vi "Cross Spectrum (Real-Im).vi"(0 "time signal X":waveform(dbl), 1 "restart averaging (F)":bool, 2 "window parameter":dbl=nan, 5 "time signal Y":waveform(dbl), 7 "window":T2=1 items=["Rectangle"=0, "Hanning"=1, "Hamming"=2, "Blackman-Harris"=3, "Exact Blackman"=4, "Blackman"=5, "Flat Top"=6, "4 Term B-Harris "=7, "7 Term B-Harris"=8, "Low Sidelobe"=9, "Blackman Nuttall"=11, "Triangle"=30, "Bartlett-Hanning"=31, "Bohman"=32, "Parzen"=33, "Welch"=34, "Kaiser"=60, "Dolph-Chebyshev"=61, "Gaussian"=62], 11 "error in (no error)":errorcluster, 12 "averaging parameters":T3={"averaging mode"=enum."No averaging", "weighting mode"=enum."Exponential", "number of averages"=10} {"number of averages" min=1}) -> (3 "averaging done":bool, 4 "real part":cluster{"f0":dbl, "df":dbl, "real part":dbl[]} {"real part" format="%.2p"; "f0" format="%0.2p"; "df" format="%0.2p"}, 6 "imaginary part":T1 {"imaginary part" format="%.2p"; "f0" format="%0.2p"; "df" format="%0.2p"}, 10 "averages completed":dbl, 15 "error out":errorcluster)   [LabVIEW 2020, in "NI_MAPro.lvlib"]
doc: "Computes the averaged cross power spectrum of the input signals. Results are returned as real and imaginary parts."
uses:
  NI_MAPro.lvlib
  windowTd.ctl
  NI_AALPro.lvlib
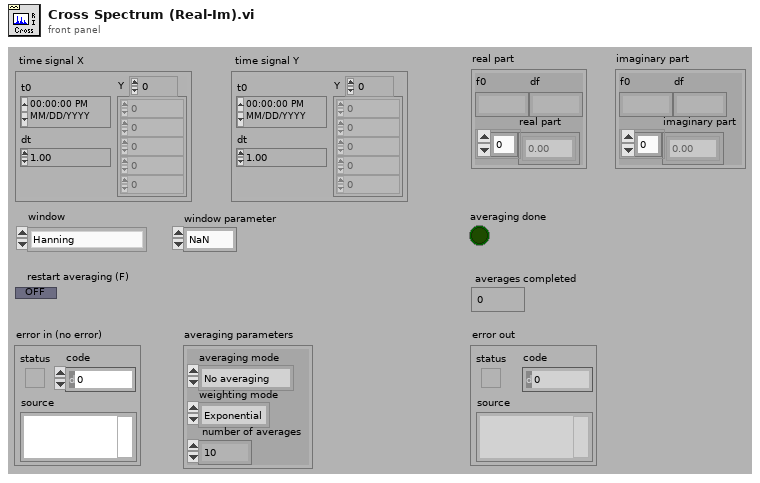
[diagram p1: front panel]
types:
  T1 = cluster{"f0":dbl, "df":dbl, "imaginary part":dbl[]}
  T2 = typedef "NI_AALPro.lvlib/windowTd.ctl" = u32
  T3 = cluster{"averaging mode":enum16{"No averaging", "Vector averaging", "RMS averaging", "Peak hold"}, "weighting mode":enum16{"Linear", "Exponential"}, "number of averages":u32}
  T4 = enum16{"No averaging", "Vector averaging", "RMS averaging", "Peak hold"}
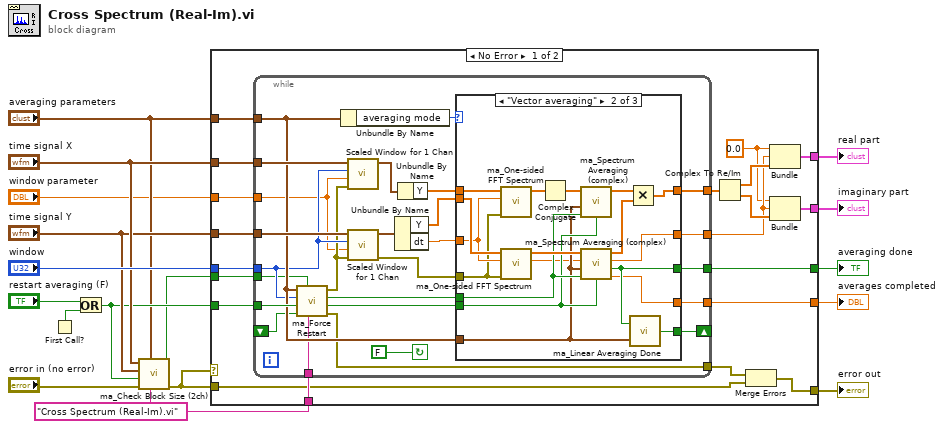
[diagram p0: block diagram]
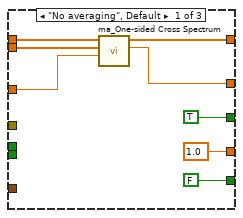
[diagram p2: hidden frame]
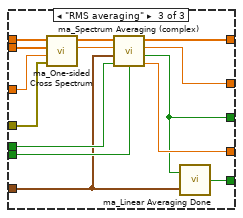
[diagram p3: hidden frame]
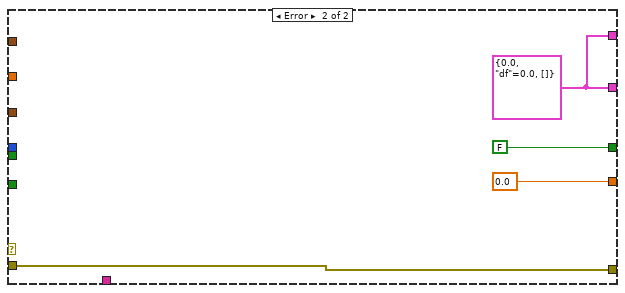
[diagram p4: hidden frame]
diagram:
  w3 = "Cross Spectrum (Real-Im).vi" ("caller VI name")
  n1 = First Call?() -> (First Call?: T/F=w7:bool)
  n2 = Or(x="restart averaging (F)", y=w7) -> (x .or. y?=w8:bool)
  n3 = call "ma_Check Block Size (2ch).vi"("caller VI name"=w3, "averaging parameters"="averaging parameters", "error in"="error in (no error)", "restart averaging (F)"=w8, "time signal Y"="time signal Y", "time signal X"="time signal X") -> ("error out"=w9:errorcluster, "force restart averaging"=w2:bool)  [unwired: 4 out]
  n4 = case shown="No Error" w9 {
    tunnel: "averaging parameters" -> [w37 _]
    tunnel: [w35 0.0 ("averages completed")] -> w17
    tunnel: "time signal X" -> [w34 _]
    tunnel: "time signal Y" -> [w33 _]
    tunnel: "window" -> [w32 _]
    tunnel: [w31 FALSE ("averaging done")] -> w15
    tunnel: w8 -> [w30 _]
    tunnel: [w23 w107] -> w14
    tunnel: w9 -> [w20 w107]
    tunnel: [w25 w104] -> w5
    tunnel: [w24 w104] -> w4
    tunnel: w3 -> [w21 _]
    tunnel: w2 -> [w19 _]
    tunnel: "window parameter" -> [w18 _]
    frame No Error {
      w26 = 0.0
      n5 = while {
        tunnel: w21 -> [w40]
        tunnel: [w41] -> w22
        tunnel: w30 -> [w55]
        shift-left: _ -> [w53]
        shift-right: [w57] -> _
        tunnel: [w58] -> w31
        tunnel: w32 -> [w45]
        tunnel: w33 -> [w59]
        tunnel: w34 -> [w60]
        tunnel: [w51] -> w27
        tunnel: [w61] -> w35
        tunnel: [w62] -> w36
        tunnel: w37 -> [w54]
        tunnel: w19 -> [w39]
        tunnel: w18 -> [w38]
        stop <- FALSE continue-if-true
        n6 = call "ma_Force Restart.vi"("caller VI name"=w40, "force restart averaging in"=w39, "linear averaging done"=w53, "restart averaging (F)"=w55, "window"=w45, "averaging parameters"=w54) -> ("error out"=w41:errorcluster, "retrieve last spectrum"=w42:bool, "force restart averaging"=w43:bool, "skip processing"=w44:errorcluster)  [unwired: 2 out]
        n7 = Unbundle By Name(w54) -> ("averaging mode"=w63:T4)
        n8 = call "Scaled Window for 1 Chan.vi"("error in (no error)"=w44, "window parameter"=w38, "window"=w45, "signal in"=w60) -> ("signal out"=w50:waveform(dbl))  [unwired: 5 in, 2 out]
        n9 = call "Scaled Window for 1 Chan.vi"("error in (no error)"=w44, "window parameter"=w38, "window"=w45, "signal in"=w59) -> ("error out"=w56:errorcluster, "signal out"=w48:waveform(dbl))  [unwired: 5 in, 1 out]
        n10 = Unbundle By Name(w48) -> ("Y"=w47:dbl[], "dt"=w46:dbl)
        n11 = Unbundle By Name(w50) -> ("Y"=w49:dbl[])
        n12 = case shown="\"Vector averaging\"" w63 {
          tunnel: w49 -> [w70 w88 w103]
          tunnel: w47 -> [w69 w86 w102]
          tunnel: w46 -> [w68 w85 w101]
          tunnel: [w66 w72 w90] -> w51
          tunnel: [w67 w89 w98] -> w62
          tunnel: w43 -> [_ w81 w99]
          tunnel: w54 -> [_ w76 w94]
          tunnel: [1.0 ("averages completed") w74 w92] -> w61
          tunnel: [TRUE ("averaging done") w75 w91] -> w58
          tunnel: [FALSE ("linear averaging done") w79 w97] -> w57
          tunnel: w56 -> [_ w78 w96]
          tunnel: w42 -> [_ w77 w95]
          frame "No averaging", Default {
            n13 = call "ma_One-sided Cross Spectrum.vi"("dt"=w68, "signal Y (V)"=w69, "signal X (V)"=w70) -> ("df"=w66:dbl, "cross spectrum (V^2 rms)"=w67:cdb[])  [unwired: 1 in, 6 out]
          }
          frame "Vector averaging" {
            n14 = call "ma_One-sided FFT Spectrum.vi"("error in"=w78, "dt"=w85, "signal (V)"=w88) -> ("FFT spectrum (Vrms)"=w87:cdb[])  [unwired: 8 out]
            n15 = call "ma_One-sided FFT Spectrum.vi"("error in"=w78, "dt"=w85, "signal (V)"=w86) -> ("df"=w73:dbl, "FFT spectrum (Vrms)"=w82:cdb[])  [unwired: 7 out]
            n16 = Complex Conjugate(1:w87) -> (0:w84:cdb[])
            n17 = call "ma_Spectrum Averaging (complex).vi"("complex spectrum"=w84, "retrieve last spectrum (F)"=w77, "averaging parameters"=w76, "restart averaging (F)"=w81) -> ("averaged complex spectrum"=w83:cdb[])  [unwired: 1 in, 4 out]
            n18 = call "ma_Spectrum Averaging (complex).vi"("complex spectrum"=w82, "df"=w73, "retrieve last spectrum (F)"=w77, "averaging parameters"=w76, "restart averaging (F)"=w81) -> ("averaged complex spectrum"=w80:cdb[], "df"=w72:dbl, "averaging done"=w75:bool, "averages completed"=w74:dbl)  [unwired: 1 out]
            n19 = Multiply(x=w83, y=w80) -> (x*y=w89:cdb[])
            n20 = call "ma_Linear Averaging Done.vi"("averaging parameters"=w76, "averaging done"=w75) -> ("linear averaging done"=w79:bool)
          }
          frame "RMS averaging" {
            n21 = call "ma_One-sided Cross Spectrum.vi"("error in"=w96, "dt"=w101, "signal Y (V)"=w102, "signal X (V)"=w103) -> ("df"=w93:dbl, "cross spectrum (V^2 rms)"=w100:cdb[])  [unwired: 6 out]
            n22 = call "ma_Spectrum Averaging (complex).vi"("complex spectrum"=w100, "df"=w93, "retrieve last spectrum (F)"=w95, "averaging parameters"=w94, "restart averaging (F)"=w99) -> ("averaged complex spectrum"=w98:cdb[], "df"=w90:dbl, "averaging done"=w91:bool, "averages completed"=w92:dbl)  [unwired: 1 out]
            n23 = call "ma_Linear Averaging Done.vi"("averaging parameters"=w94, "averaging done"=w91) -> ("linear averaging done"=w97:bool)
          }
        }
      }
      n24 = Complex To Re/Im(x + iy=w36) -> (x=w29:dbl[], y=w28:dbl[])
      n25 = Merge Errors(w22, w20) -> (w23:errorcluster)
      n26 = Bundle(w26, "df"=w27, w29) -> (w25:cluster{dbl, "df":dbl, dbl[]})  [unwired: 1 out]
      n27 = Bundle(w26, "df"=w27, w28) -> (w24:cluster{dbl, "df":dbl, dbl[]})  [unwired: 1 out]
    }
    frame Error {
      w104 = cluster{dbl, "df":dbl, dbl[]} {0.0, "df"=0.0, []}
    }
  }
  "averages completed" <- w17
  "error out" <- w14
  "averaging done" <- w15
  "real part" <- w5
  "imaginary part" <- w4
